vi "compare_item.vi"(5 "item":string[](array[string]), 7 "folders":string[](array[string]), 8 "filenames":string[](array[string]), 9 "start path":path) -> (0 "exist":bool, 1 "folders 2":string[](array[string]), 2 "filenames 2":string[](array[string]), 3 "item 2":string[](array[string]), 4 "modified":bool)   [LabVIEW 2010]
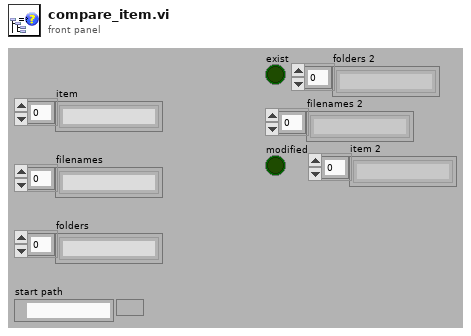
[diagram p1: front panel]
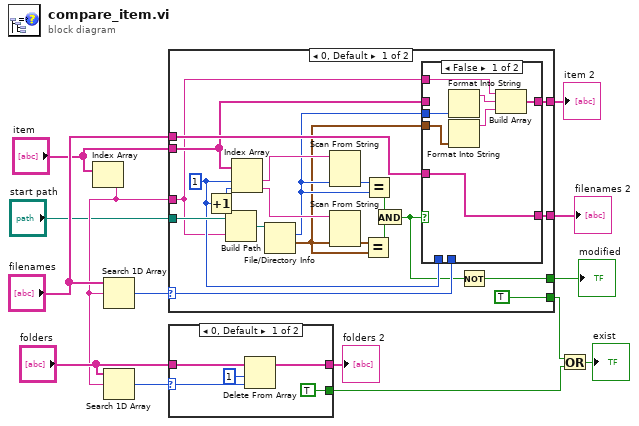
[diagram p0: block diagram]
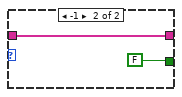
[diagram p2: hidden frame]
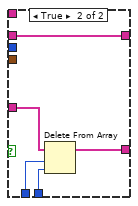
[diagram p3: hidden frame]
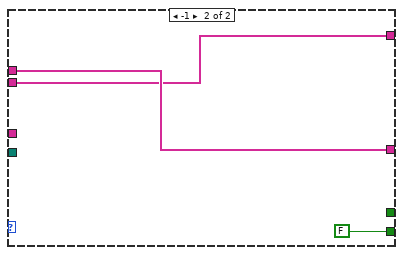
[diagram p4: hidden frame]
diagram:
  n1 = Index Array(array="item") -> (element=w10:string)  [unwired: 1 in]
  n2 = Search 1D Array(1D array="filenames", element=w10) -> (index of element=w8:i32)  [unwired: 1 in]
  n3 = Search 1D Array(1D array="folders", element=w10) -> (index of element=w13:i32)  [unwired: 1 in]
  n4 = case shown="0, Default" w8 {
    selector: w8 -> [w25 _]
    tunnel: "start path" -> [w35 _]
    tunnel: w10 -> [w15 _]
    tunnel: "item" -> [w16 w48]
    tunnel: "filenames" -> [w24 w50]
    tunnel: [w23 w50] -> w3
    tunnel: [TRUE FALSE] -> w7
    tunnel: [w20 _] -> w2
    tunnel: [w17 w48] -> w1
    frame 0, Default {
      w26 = 1 ("index")
      n5 = Increment(x=w26) -> (x+1=w33:i32)
      n6 = Build Path(base path=w35, name or relative path=w15) -> (appended path=w34:path)
      n7 = Index Array(array=w16, index #1=w26, index #2=w33) -> (element #1=w32:string, element #2=w31:string)
      n8 = File/Directory Info(path=w34) -> (size=w19:i64, last mod=w18:timestamp)  [unwired: 1 in, 5 out]
      n9 = Scan From String(input string=w32, default 1=w19) -> (output 1=w30:i64)  [unwired: 3 in, 3 out]
      n10 = Scan From String(input string=w31, default 1=w18) -> (output 1=w29:timestamp)  [unwired: 3 in, 3 out]
      n11 = Equal?(x=w29, y=w18) -> (x = y?=w28:bool)
      n12 = Equal?(x=w30, y=w19) -> (x = y?=w27:bool)
      n13 = And(x=w27, y=w28) -> (x .and. y?=w22:bool)
      n14 = case shown="False" w22 {
        tunnel: w26 -> [_ w47]
        tunnel: w25 -> [_ w46]
        tunnel: w24 -> [w42 w45]
        tunnel: [w42 w44] -> w23
        tunnel: w19 -> [w41 _]
        tunnel: w18 -> [w40 _]
        tunnel: [w37 w43] -> w17
        tunnel: w16 -> [_ w43]
        tunnel: w15 -> [w36 _]
        frame False {
          n15 = Format Into String(w41) -> (resulting string=w39:string)  [unwired: 3 in, 1 out]
          n16 = Format Into String(w40) -> (resulting string=w38:string)  [unwired: 3 in, 1 out]
          n17 = Build Array(w36, w39, w38) -> (w37:string[])
        }
        frame True {
          n18 = Delete From Array(array=w45, length=w47, index=w46) -> (array with subset deleted=w44:string[])  [unwired: 1 out]
        }
      }
      n19 = Not(x=w22) -> (.not. x?=w20:bool)
    }
    frame -1 {
    }
  }
  "filenames 2" <- w3
  "modified" <- w2
  "item 2" <- w1
  n20 = case shown="0, Default" w13 {
    selector: w13 -> [w55 _]
    tunnel: "folders" -> [w53 w57]
    tunnel: [w52 w57] -> w4
    tunnel: [TRUE FALSE] -> w6
    frame 0, Default {
      n21 = Delete From Array(array=w53, length=1, index=w55) -> (array with subset deleted=w52:string[])  [unwired: 1 out]
    }
    frame -1 {
    }
  }
  "folders 2" <- w4
  n22 = Or(x=w7, y=w6) -> (x .or. y?=→"exist":bool)
